vi "(Depricated) Set Storage Line Color.vi"(8 "error in (no error)":errorcluster, 9 "Bit Field":u16, 10 "Round Color Box":u32(colorbox), 11 "AMS Gas in":refnum<class "AMS Gas.lvclass">) -> (0 "error out":errorcluster, 3 "AMS Gas out":refnum<class "AMS Gas.lvclass">)   [LabVIEW 2015, in "AMS UI.lvlib" / "AMS Gas.lvclass"]
uses:
  AMS Gas.lvclass
  AMS Gas.lvclass/AMS Gas.ctl
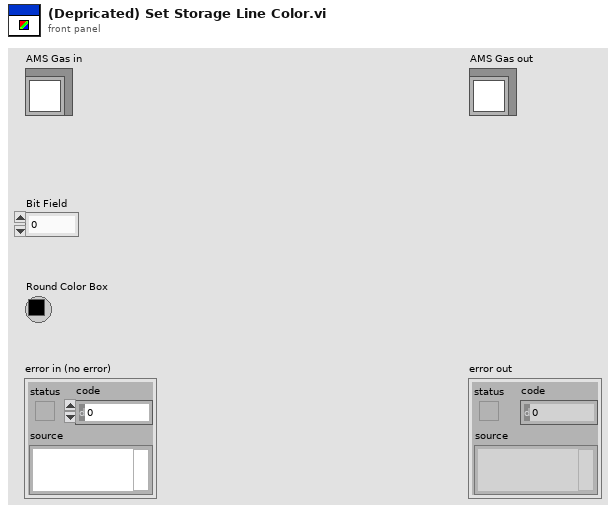
[diagram p1: front panel]
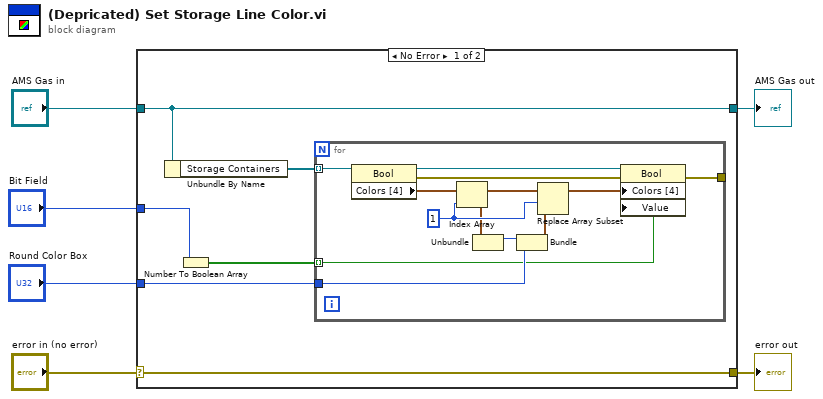
[diagram p0: block diagram]
diagram:
  n1 = case shown="No Error" "error in (no error)" {
    selector: "error in (no error)" -> [w12 w26]
    tunnel: [w12 w26] -> w5
    tunnel: [w11 w25] -> w3
    tunnel: "AMS Gas in" -> [w11 w25]
    tunnel: "Round Color Box" -> [w9 _]
    tunnel: "Bit Field" -> [w8 _]
    frame No Error {
      n2 = Unbundle By Name(w11) -> ("Storage Containers"=w10:refnum<vi>[])
      n3 = Number To Boolean Array(number=w8) -> (Boolean array=w7:bool[])
      n4 = for {
        tunnel: w10 -> [w24] mode=indexing
        tunnel: w9 -> [w20]
        tunnel: [w21] -> _
        tunnel: w7 -> [w13] mode=indexing
        w18 = 1 ("index")
        n5 = property class="Bool"(reference=w24) -> (reference out=w23:refnum<vi>, error out=w22:errorcluster, "Colors [4]"=w19:cluster{u32, u32}[])  [unwired: 1 in]
        n6 = Index Array(array=w19, index=w18) -> (element=w14:cluster{u32, u32})
        n7 = Unbundle(w14) -> (w15:u32)  [unwired: 1 out]
        n8 = Bundle(w15, "Round Color Box"=w20) -> (w17:cluster{u32, "Round Color Box":u32})  [unwired: 1 in]
        n9 = Replace Array Subset(array=w19, new element=w17, index=w18) -> (w16:cluster{u32, u32}[])
        n10 = property class="Bool"(reference=w23, error in=w22, "Colors [4]"=w16, "Value"=w13) -> (error out=w21:errorcluster)  [unwired: 1 out]
      }
    }
    frame Error {
    }
  }
  "error out" <- w5
  "AMS Gas out" <- w3
